vi "Running_Ch_Average.vi"(4 "Shift In":dbl[](array[numeric]), 5 "History length":i32=10, 6 "Reset Average after Seconds":dbl=120.0, 7 "New Value":dbl) -> (0 "Shift Out":dbl[](array[numeric]), 3 "mean":dbl format="%0.2f")   [LabVIEW 2016]
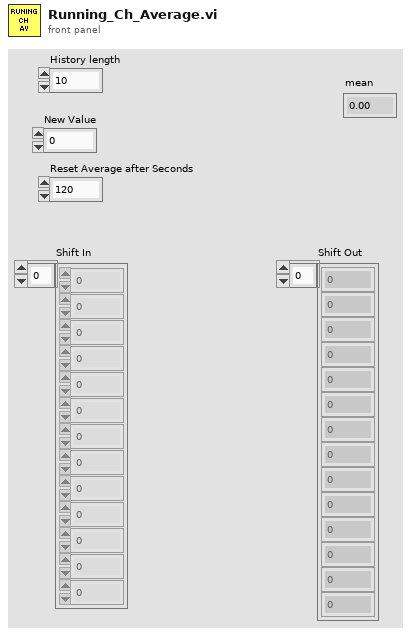
[diagram p1: front panel]
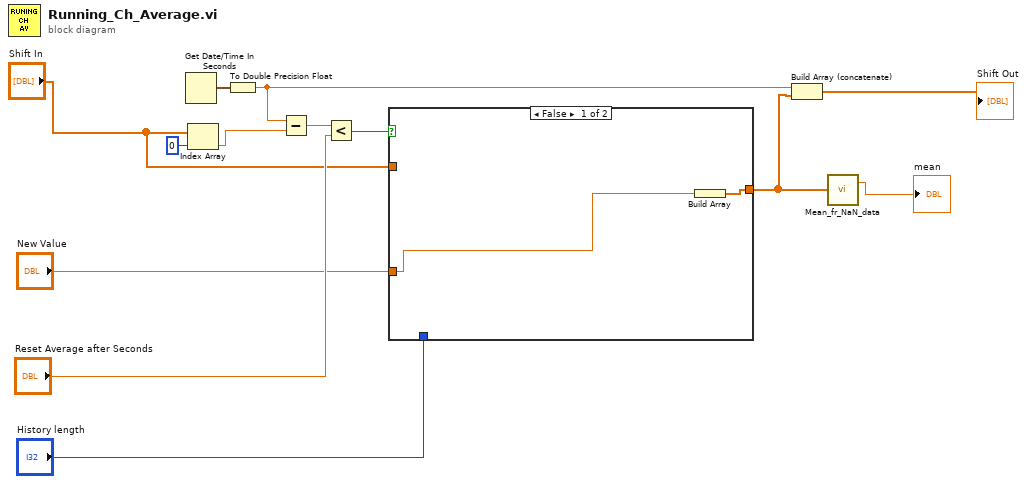
[diagram p0: block diagram]
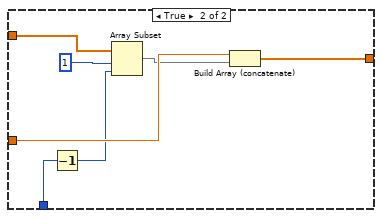
[diagram p2: hidden frame]
diagram:
  n1 = Get Date/Time In Seconds() -> (seconds since 1Jan1904=w12:timestamp)
  n2 = Index Array(array="Shift In", index=0) -> (element=w10:dbl)
  n3 = To Double Precision Float(number=w12) -> (double precision float=w11:dbl)
  n4 = Subtract(x=w11, y=w10) -> (x-y=w9:dbl)
  n5 = Less?(x=w9, y="Reset Average after Seconds") -> (x < y?=w7:bool)
  n6 = case shown="False" w7 {
    tunnel: "Shift In" -> [_ w22]
    tunnel: "New Value" -> [w15 w20]
    tunnel: [w14 w18] -> w2
    tunnel: "History length" -> [_ w17]
    frame False {
      n7 = Build Array(w15) -> (w14:dbl[])
    }
    frame True {
      n8 = Decrement(x=w17) -> (x-1=w16:i32)
      n9 = Array Subset(array=w22, index=1, length=w16) -> (w19:dbl[])
      n10 = Build Array (concatenate)(w20, w19) -> (w18:dbl[])
    }
  }
  n11 = Build Array (concatenate)(w11, w2) -> (→"Shift Out":dbl[])
  n12 = call "Mean_fr_NaN_data.vi"("Data"=w2) -> ("Mean value"=→"mean":dbl)  [unwired: 1 out]
